vi "Create Results Folder Path.vi"(10 "CurrentProductNum":string, 11 "StationName":string) -> (3 "Folder path":path)   [LabVIEW 2021, in "SQLite.lvclass"]
uses:
  SQLite.lvclass
  SQLite.lvclass/SQLite.ctl
  <userlib>/sushu/sushu.lvlib
  vi.lib_New/TopPath/TopPath.lvlib
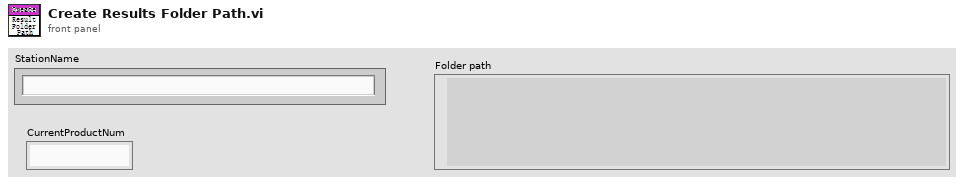
[diagram p1: front panel]
types:
  T1 = typedef "TopPath.lvlib/Top Path.ctl" = cluster{"LV Source":path, "FilePath":path, "Data":path}
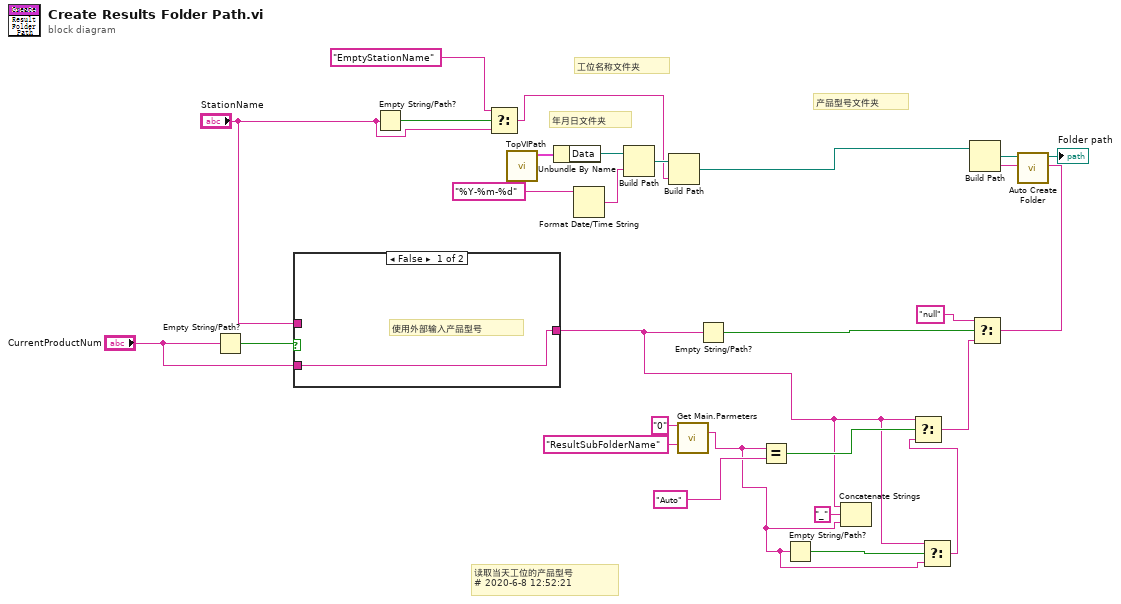
[diagram p0: block diagram]
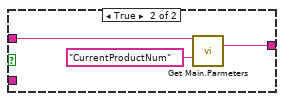
[diagram p2: hidden frame]
diagram:
  # "读取当天工位的产品型号\n# 2020-6-8 12:52:21"
  # "产品型号文件夹"
  # "工位名称文件夹"
  # "年月日文件夹"
  n1 = Empty String/Path?(string/path="CurrentProductNum") -> (empty?=w2:bool)
  n2 = case shown="False" w2 {
    tunnel: "StationName" -> [_ w30]
    tunnel: [w28 w29] -> w5
    tunnel: "CurrentProductNum" -> [w28 _]
    frame False {
      # "使用外部输入产品型号"
    }
    frame True {
      n3 = call "Get Main.Parmeters.vi"("Main"=w30, "VariableName"="CurrentProductNum") -> ("Value"=w29:string)  [unwired: 6 in, 7 out]
    }
  }
  n4 = Empty String/Path?(string/path="StationName") -> (empty?=w16:bool)
  n5 = Select(t="EmptyStationName", s=w16, f="StationName") -> (s? t:f=w13:string)
  n6 = call "TopVIPath.vi"() -> ("TopPath"=w27:T1)  [unwired: 10 in, 1 out]
  n7 = Unbundle By Name(w27) -> ("Data"=w23:path)
  n8 = Format Date/Time String(time format string (%c)="%Y-%m-%d") -> (date/time string=w25:string)  [unwired: 2 in]
  n9 = Build Path(base path=w23, name or relative path=w25) -> (appended path=w24:path)
  n10 = Build Path(base path=w24, name or relative path=w13) -> (appended path=w22:path)
  n11 = call "Get Main.Parmeters.vi"("Main"="0", "VariableName"="ResultSubFolderName") -> ("Value"=w4:string)  [unwired: 6 in, 7 out]
  n12 = Empty String/Path?(string/path=w5) -> (empty?=w18:bool)
  n13 = Equal?(x=w4, y="Auto") -> (x = y?=w9:bool)
  n14 = Empty String/Path?(string/path=w4) -> (empty?=w6:bool)
  n15 = Concatenate Strings(w5, "_" ("string"), w4) -> ()  [unwired: 1 out]
  n16 = Select(t=w5, s=w6, f=w4) -> (s? t:f=w3:string)
  n17 = Select(t=w5, s=w9, f=w3) -> (s? t:f=w8:string)
  n18 = Select(t="null", s=w18, f=w8) -> (s? t:f=w20:string)
  n19 = Build Path(base path=w22, name or relative path=w20) -> (appended path=w21:path)
  n20 = call <userlib>:"Auto Create Folder.vi"("Folder path"=w21) -> ("Folder path"=→"Folder path":path)  [unwired: 9 in, 1 out]
